vi "Initialize.vi"(8 "error in (no error)":errorcluster, 11 "DB in":refnum<class "DB.lvclass">) -> (0 "error out":errorcluster, 3 "DB out":refnum<class "DB.lvclass">)   [LabVIEW 2018, in "DB.lvclass"]
uses:
  DB.lvclass
  C:/Users/Sergey Denisov/Documents/REPS/TRANCON/Classes/GeneralFunctionality/GeneralFunctionality.lvclass
  GeneralFunctionality/GeneralFunctionality.lvclass/GeneralFunctionality.ctl
  GeneralFunctionality/GeneralFunctionality.lvclass
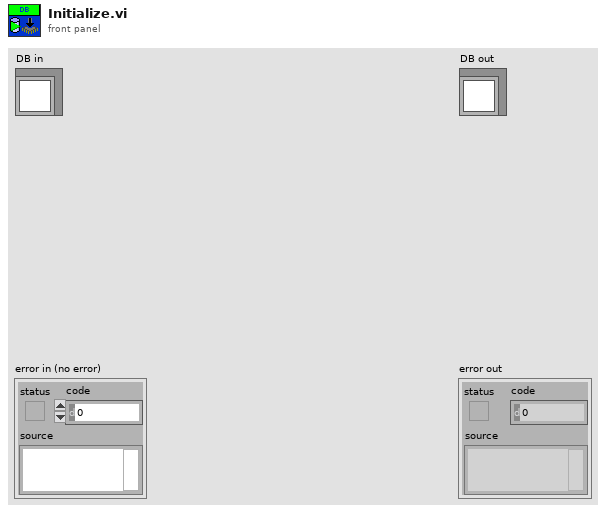
[diagram p1: front panel]
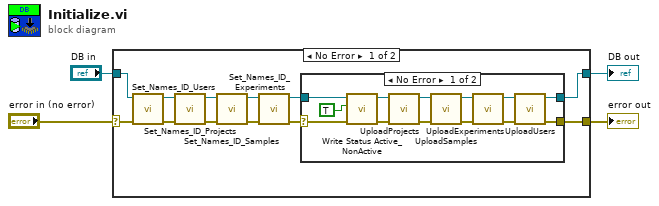
[diagram p0: block diagram]
diagram:
  n1 = case shown="No Error" "error in (no error)" {
    selector: "error in (no error)" -> [w7 w33]
    tunnel: [w16 w33] -> w3
    tunnel: [w15 w32] -> w1
    tunnel: "DB in" -> [w10 w32]
    frame No Error {
      n2 = call "Set_Names_ID_Users.vi"("error in (no error)"=w7, "DB in"=w10) -> ("error out"=w5:errorcluster, "DB out"=w9:refnum<class "DB.lvclass">)  [unwired: 8 in]
      n3 = call "Set_Names_ID_Projects.vi"("error in (no error)"=w5, "DB in"=w9) -> ("error out"=w13:errorcluster, "DB out"=w14:refnum<class "DB.lvclass">)  [unwired: 8 in]
      n4 = call "Set_Names_ID_Samples.vi"("error in (no error)"=w13, "DB in"=w14) -> ("error out"=w11:errorcluster, "DB out"=w12:refnum<class "DB.lvclass">)  [unwired: 8 in]
      n5 = call "Set_Names_ID_Experiments.vi"("error in (no error)"=w11, "DB in"=w12) -> ("error out"=w6:errorcluster, "DB out"=w8:refnum<class "DB.lvclass">)  [unwired: 8 in]
      n6 = case shown="No Error" w6 {
        selector: w6 -> [w28 w30]
        tunnel: w8 -> [w27 w31]
        tunnel: [w18 w31] -> w15
        tunnel: [w19 w30] -> w16
        frame No Error {
          n7 = call "Write Status Active_NonActive.vi"("error in (no error)"=w28, "Status Active/NonActive"=TRUE, "GeneralFunctionality in"=w27) -> ("error out"=w25:errorcluster, "GeneralFunctionality out"=w26:refnum<class "DB.lvclass">)  [unwired: 7 in]
          n8 = call "UploadProjects.vi"("error in (no error)"=w25, "DB in"=w26) -> ("error out"=w24:errorcluster, "DB out"=w23:refnum<class "DB.lvclass">)  [unwired: 8 in]
          n9 = call "UploadSamples.vi"("error in (no error)"=w24, "DB in"=w23) -> ("error out"=w22:errorcluster, "DB out"=w21:refnum<class "DB.lvclass">)  [unwired: 8 in]
          n10 = call "UploadExperiments.vi"("error in (no error)"=w22, "DB in"=w21) -> ("error out"=w20:errorcluster, "DB out"=w17:refnum<class "DB.lvclass">)  [unwired: 8 in]
          n11 = call "UploadUsers.vi"("error in (no error)"=w20, "DB in"=w17) -> ("error out"=w19:errorcluster, "DB out"=w18:refnum<class "DB.lvclass">)  [unwired: 8 in]
        }
        frame Error {
        }
      }
    }
    frame Error {
    }
  }
  "error out" <- w3
  "DB out" <- w1
